vi "Configure Port Power.vi"(7 "Maximum Power Limit (0)":dbl, 8 "error in (no error)":errorcluster, 9 "Port (1)":i32=1, 10 "Enable Power Limit (F: Disabled)":bool, 11 "VISA resource name":refnum<visa-resource-name>) -> (0 "error out":errorcluster, 3 "VISA resource name out":refnum<visa-resource-name>)   [LabVIEW 2022 SP3, in "Agilent ENA Series.lvlib"]
doc: "Configures the power limit that can come from the specified port.\n\nNote:\nValid for E5072A only."
uses:
  <instrlib>/Agilent ENA Series/Agilent ENA Series.lvlib
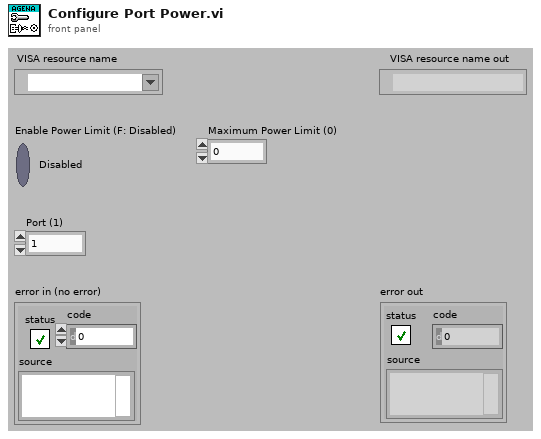
[diagram p1: front panel]
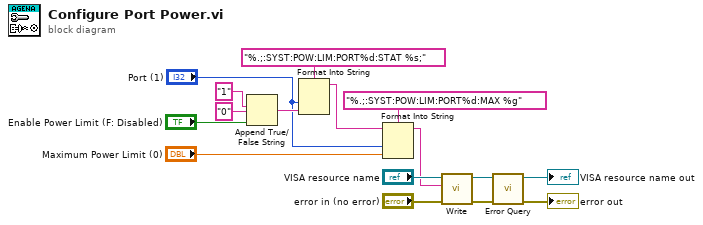
[diagram p0: block diagram]
diagram:
  n1 = Append True/False String(1:"Enable Power Limit (F: Disabled)", 2:"0" ("true string"), 3:"1" ("true string")) -> (0:w6:string)  [unwired: 1 in]
  n2 = Format Into String(format string="%.;:SYST:POW:LIM:PORT%d:STAT %s;", "Port (1)", w6) -> (resulting string=w2:string)  [unwired: 2 in, 1 out]
  n3 = Format Into String(format string="%.;:SYST:POW:LIM:PORT%d:MAX %g", initial string=w2, "Port (1)", "Maximum Power Limit (0)") -> (resulting string=w1:string)  [unwired: 1 in, 1 out]
  n4 = call <instrlib>:"Write.vi"("error in (no error)"="error in (no error)", "String ()"=w1, "VISA resource name"="VISA resource name") -> ("error out"=w14:errorcluster, "VISA resource name out"=w13:refnum<visa-resource-name>)  [unwired: 6 in, 1 out]
  n5 = call <instrlib>:"Error Query.vi"("error in (no error)"=w14, "VISA resource name"=w13) -> ("error out"=→"error out":errorcluster, "VISA resource name out"=→"VISA resource name out":refnum<visa-resource-name>)  [unwired: 6 in, 2 out]
